vi "Disconnect.vi"(10 "error in (no error)":errorcluster, 11 "WAMP Client in":refnum<class "WAMP Client.lvclass">) -> (2 "error out":errorcluster, 3 "WAMP Client out":refnum<class "WAMP Client.lvclass">)   [LabVIEW 2020, in "wamplv.lvlib" / "WAMP Client.lvclass"]
uses:
  <userlib>/wamplv/WAMP Client/WAMP Client.lvclass
  <userlib>/wamplv/WAMP Client/WAMP Client.lvclass/WAMP Client.ctl
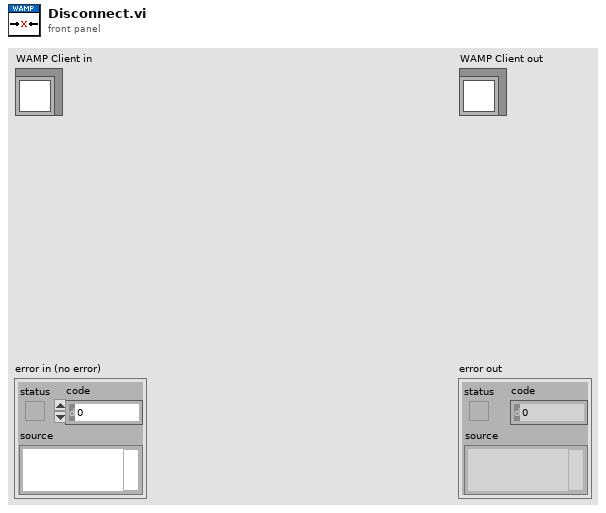
[diagram p1: front panel]
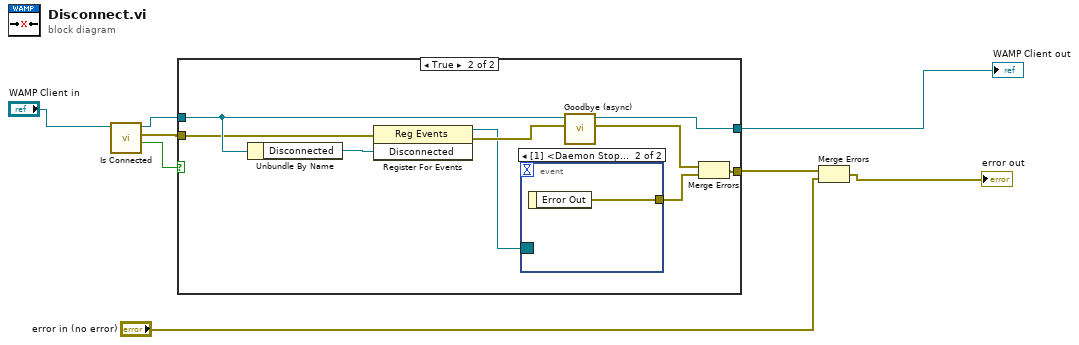
[diagram p0: block diagram]
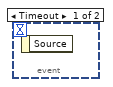
[diagram p3: hidden frame]
diagram:
  n1 = call-dynamic "Is Connected.vi"("WAMP Client in"="WAMP Client in") -> ("Is Connected?"=w7:bool, "error out"=w4:errorcluster, "WAMP Client out"=w5:refnum<class "WAMP Client.lvclass">)  [unwired: 8 in]
  n2 = case shown="True" w7 {
    tunnel: [w10 w19] -> w6
    tunnel: w5 -> [w10 w16]
    tunnel: w4 -> [w9 w11]
    tunnel: [w9 w18] -> w2
    frame False {
    }
    frame True {
      n3 = Unbundle By Name(w16) -> ("Disconnected"=w15:refnum<user-event>)
      n4 = register-events(error in=w11, w15) -> (reference out=w13:refnum<event-registration>, error out=w14:errorcluster)  [unwired: 1 in]
      n5 = event shown="[1] <Daemon Stopped>: User Event" {
        selector: w13 -> [_ _]
        dyn-events: _ -> [_ _]
        timeout: _ -> [_ _]
        tunnel: [_ w20] -> w12
        event Timeout {
          n6 = event-data() -> ()  [unwired: 1 in, 1 out]
        }
        event User Event {
          n7 = event-data() -> ("Error Out"=w20:errorcluster)  [unwired: 1 in]
        }
      }
      n8 = call-dynamic "Goodbye (async).vi"("error in (no error)"=w14, "WAMP Client in"=w16) -> ("error out"=w17:errorcluster, "WAMP Client out"=w19:refnum<class "WAMP Client.lvclass">)  [unwired: 8 in]
      n9 = Merge Errors(w17, w12) -> (w18:errorcluster)
    }
  }
  "WAMP Client out" <- w6
  n10 = Merge Errors(w2, "error in (no error)") -> (→"error out":errorcluster)
